vi "Read Time.vi"(8 "error in (no error)":errorcluster, 11 "Nested Value Update Msg in":refnum<class "Nested Value Update Msg.lvclass">) -> (0 "error out":errorcluster, 2 "Time":u32, 3 "Nested Value Update Msg out":refnum<class "Nested Value Update Msg.lvclass">)   [LabVIEW 2020, in "MVA Framework.lvlib" / "IViewable.lvlib" / "Nested Value Update Msg.lvclass"]
uses:
  Nested Value Update Msg.lvclass
  Nested Value Update Msg.lvclass/Nested Value Update Msg.ctl
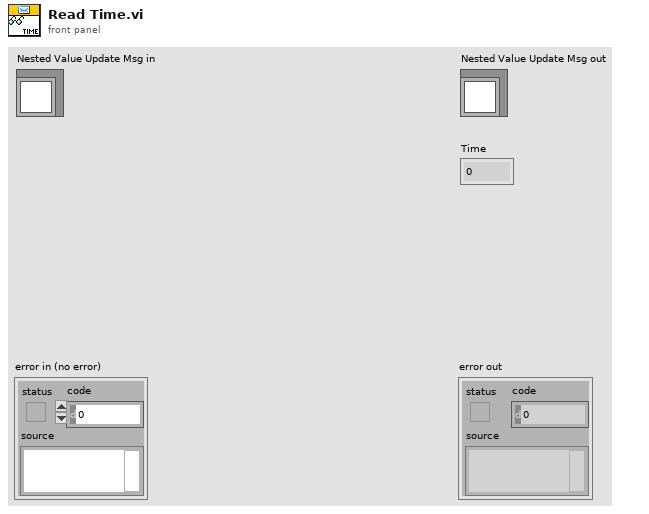
[diagram p1: front panel]
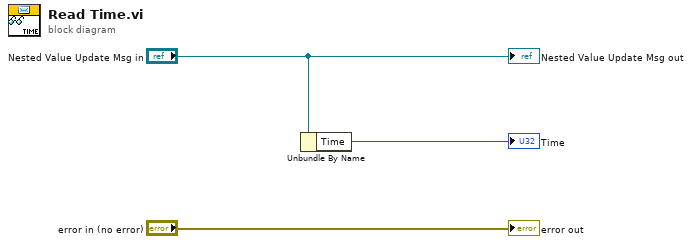
[diagram p0: block diagram]
diagram:
  n1 = Unbundle By Name("Nested Value Update Msg in") -> ("Time"=→"Time":u32)
  "error out" <- "error in (no error)"
  "Nested Value Update Msg out" <- "Nested Value Update Msg in"
